vi "Inner_SubVI_Byte47_60 (SubVI).vi"(7 "Numeric in":u16) -> (0 "Beta Version":u16, 1 "Bugfix Version":u16, 2 "Minor Version":u16, 3 "Major Version":u16)   [LabVIEW 2024]
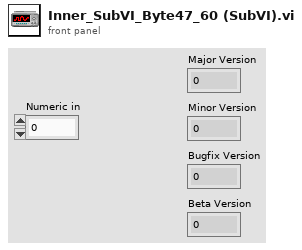
[diagram p1: front panel]
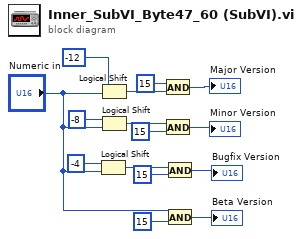
[diagram p0: block diagram]
diagram:
  n1 = Logical Shift(y=i16 -4, x="Numeric in") -> (x << y=w8:u16)
  n2 = Logical Shift(y=i16 -12, x="Numeric in") -> (x << y=w2:u16)
  n3 = Logical Shift(y=i16 -8, x="Numeric in") -> (x << y=w5:u16)
  n4 = And(x=u16 15, y=w2) -> (x .and. y?=→"Major Version":u16)
  n5 = And(x=w5, y=u16 15) -> (x .and. y?=→"Minor Version":u16)
  n6 = And(x=w8, y=u16 15) -> (x .and. y?=→"Bugfix Version":u16)
  n7 = And(x="Numeric in", y=u16 15) -> (x .and. y?=→"Beta Version":u16)
